vi "LoadAdditionalData.vi"(8 "error in (no error)":errorcluster, 11 "DigitalOutput_Simulation In":refnum<class "TesteractHAL_DigitalOutput_Simulation.lvclass">) -> (0 "error out":errorcluster, 3 "DigitalOutput_Simulation Out":refnum<class "TesteractHAL_DigitalOutput_Simulation.lvclass">)   [LabVIEW 2017, in "TesteractHAL_DigitalOutput_Simulation.lvlib" / "TesteractHAL_DigitalOutput_Simulation.lvclass"]
uses:
  TesteractHAL_DigitalOutput_Simulation.lvclass
  C:/Program Files (x86)/Testeract/HWLib/HAL/Device/TesteractHAL_Device.lvlibp/TesteractHAL_Device.lvclass
  TesteractHAL_DigitalOutput_Simulation.lvclass/TesteractHAL_DigitalOutput_Simulation.ctl
  Program Files (x86)/Testeract/HWLib/HAL/Device/TesteractHAL_Device.lvlibp/ReadDeviceName.vi
  Program Files (x86)/Testeract/HWLib/HAL/DeviceCfg/TesteractHAL_DeviceCfg_API.lvlibp
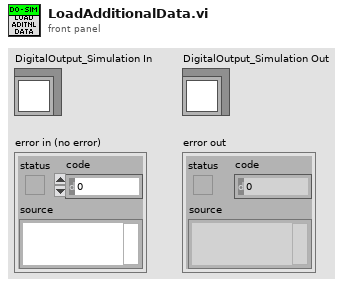
[diagram p1: front panel]
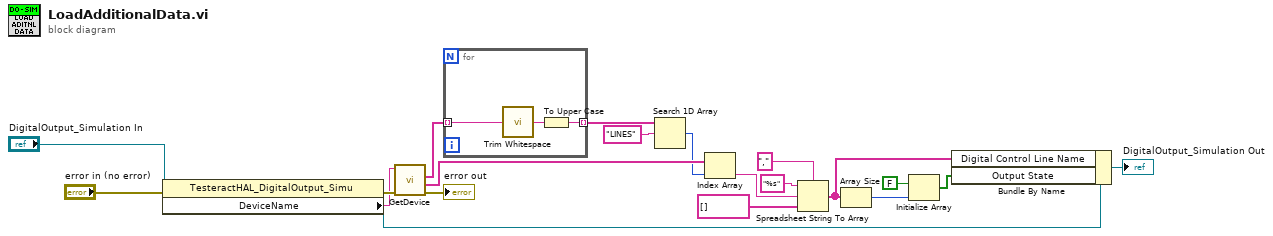
[diagram p0: block diagram]
diagram:
  n1 = property class="TesteractHAL_DigitalOutput_Simu"(reference="DigitalOutput_Simulation In", error in="error in (no error)") -> (reference out=w15:refnum<class "TesteractHAL_DigitalOutput_Simulation.lvclass">, error out=w20:errorcluster, "DeviceName"=w19:string)
  n2 = call "GetDevice.vi"("error in (no error)"=w20, "Device"=w19) -> ("error out"=→"error out":errorcluster, "Values"=w18:string[], "Keys"=w16:string[])  [unwired: 6 in, 1 out]
  n3 = for {
    tunnel: [w23] -> w17 mode=indexing
    tunnel: w16 -> [w22] mode=indexing
    n4 = call <vilib>:"Trim Whitespace.vi"("string"=w22) -> ("trimmed string"=w21:string)  [unwired: 1 in]
    n5 = To Upper Case(1:w21) -> (0:w23:string)
  }
  n6 = Search 1D Array(1D array=w17, element="LINES") -> (index of element=w10:i32)  [unwired: 1 in]
  n7 = Index Array(array=w18, index=w10) -> (element=w9:string)
  n8 = Spreadsheet String To Array(delimiter (Tab)=",", format string="%s", spreadsheet string=w9, array type (2D Dbl)=string[] []) -> (array=w4:string[])
  n9 = Array Size(array=w4) -> (size(s)=w3:i32)
  n10 = Initialize Array(FALSE ("Output State"), w3) -> (w1:bool[])
  n11 = Bundle By Name(cluster=w15, "Digital Control Line Name"=w4, "Output State"=w1) -> (→"DigitalOutput_Simulation Out":refnum<class "TesteractHAL_DigitalOutput_Simulation.lvclass">)
